vi "Edge Counter.vi"() -> ()   [LabVIEW 2017]
panel:
  out "Seatbelt Velocity":dbl
  out "Rising Edge?":bool
  out "Edge Counter":dbl
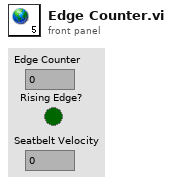
[diagram p1: front panel]
diagram:
